vi "Get LVClass Control Reference.vi"(0 "VI in":refnum<vi>, 5 "name/order":string, 11 "error in (no error)":errorcluster) -> (4 "Cluster out":refnum<vi>, 15 "error out":errorcluster)   [LabVIEW 2021, in "Migrator Reusables.lvlib"]
uses:
  Migrator Reusables.lvlib
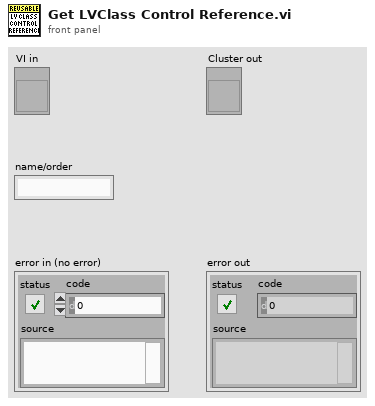
[diagram p1: front panel]
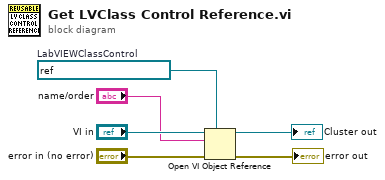
[diagram p0: block diagram]
diagram:
  w1 = refnum<vi> refnum  # LabVIEWClassControl
  n1 = Open VI Object Reference(7:w1, 8:"error in (no error)", 10:"name/order", 11:"VI in") -> (0:→"error out":errorcluster, 3:→"Cluster out":refnum<vi>)
